vi "Init.vi"(6 "Teller":refnum<class "Teller.lvclass">, 9 "Error":errorcluster, 10 "Actor":refnum<class "Actor.lvclass">) -> (3 "Terminate Msg out":refnum<class "Terminate Msg.lvclass">)   [LabVIEW 2025, in "jettl.lvlib" / "Terminate Msg.lvlib" / "Terminate Msg.lvclass"]
uses:
  Terminate Msg.lvclass
  Terminate Msg.lvclass/Terminate Msg.ctl
  Actor/Actor/Actor.lvclass
  Teller/Teller/Teller.lvclass
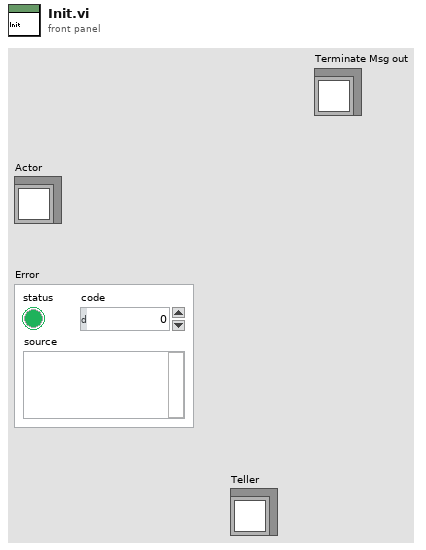
[diagram p1: front panel]
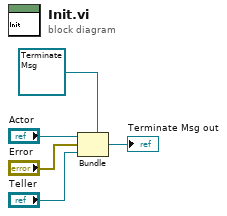
[diagram p0: block diagram]
diagram:
  n1 = Bundle "Bundle"(cluster=refnum<class "Terminate Msg.lvclass"> refnum ("Last Ack Creator Queue Msg Strategy out"), "Actor", "Error", "Teller") -> (→"Terminate Msg out":refnum<class "Terminate Msg.lvclass">)
